vi "LHF.DB.Mongo.Server.GetDatabase.vi"(0 "MongoServer in":refnum<k24>, 2 "name":string, 5 "error in (no error)":errorcluster) -> (14 "MongoServer":refnum<k24>, 15 "MongoDatabase":refnum<k24>, 19 "error out":errorcluster)   [LabVIEW 2013, in "LHF.DB.Mongo.lvclass"]
uses:
  LHF.DB.Mongo.lvclass
  C:/Users/Ricardo/Desktop/Projetos/LabVIEW-MongoDB/src/Driver/MongoDB.Driver.dll
  LabVIEW-MongoDB/src/Driver/MongoDB.Driver.dll
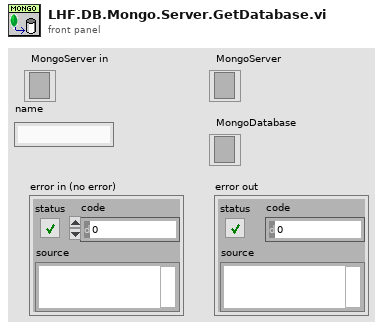
[diagram p1: front panel]
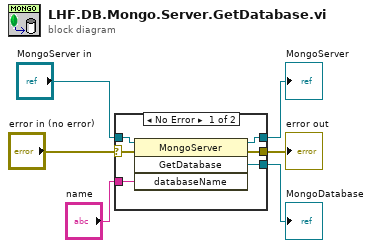
[diagram p0: block diagram]
diagram:
  n1 = case shown="No Error" "error in (no error)" {
    selector: "error in (no error)" -> [w8 w13]
    tunnel: [w12 _] -> w6
    tunnel: [w11 w14] -> w5
    tunnel: "MongoServer in" -> [w10 w14]
    tunnel: "name" -> [w9 _]
    tunnel: [w7 w13] -> w1
    frame No Error {
      n2 = invoke class="MongoServer" method="GetDatabase"(reference=w10, error in=w8, "databaseName"=w9) -> (reference out=w11:refnum<k24>, error out=w7:errorcluster, "GetDatabase"=w12:refnum<k24>)  [unwired: 1 in, 1 out]
    }
    frame Error {
    }
  }
  "error out" <- w1
  "MongoDatabase" <- w6
  "MongoServer" <- w5
